vi "AnalyzeCommonTypeDefCallers.vi"() -> ()   [LabVIEW 2013, in "DiscoverCommonTypeDefCallers.lvlib"]
uses:
  DiscoverCommonTypeDefCallers.lvlib
panel:
  in  "Tab Control":enum32{"Tree View", "Table View"}(tab)
  in  "Dependent TypeDefs (Tree)":string(tree) caption="Dependent TypeDefs"
  out "Dependent TypeDefs (table)":string[][](table) caption="Dependent TypeDefs"
  in  "Application Reference":refnum<vi>
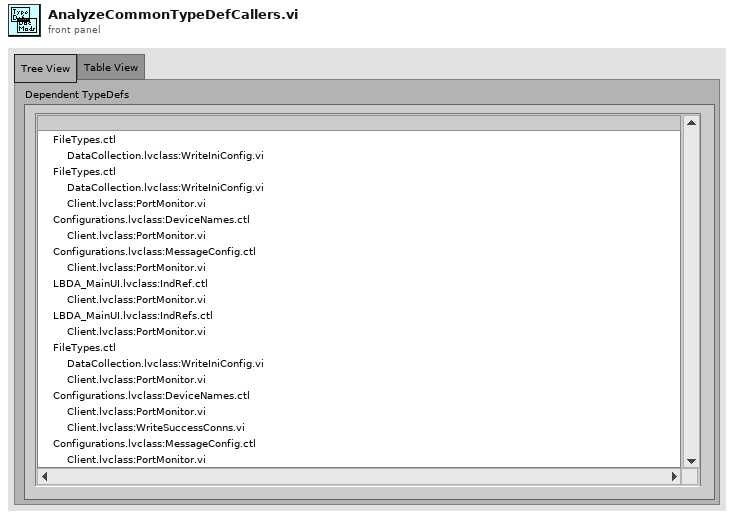
[diagram p1: front panel]
types:
  T1 = typedef "DiscoverCommonTypeDefCallers.lvlib/DependendentTypeDefwParents.ctl" = cluster{"TypeDef":string, "Non-strict / Strict":enum32{"Non-strict", "Strict"}, "Parent VIs":string[]}
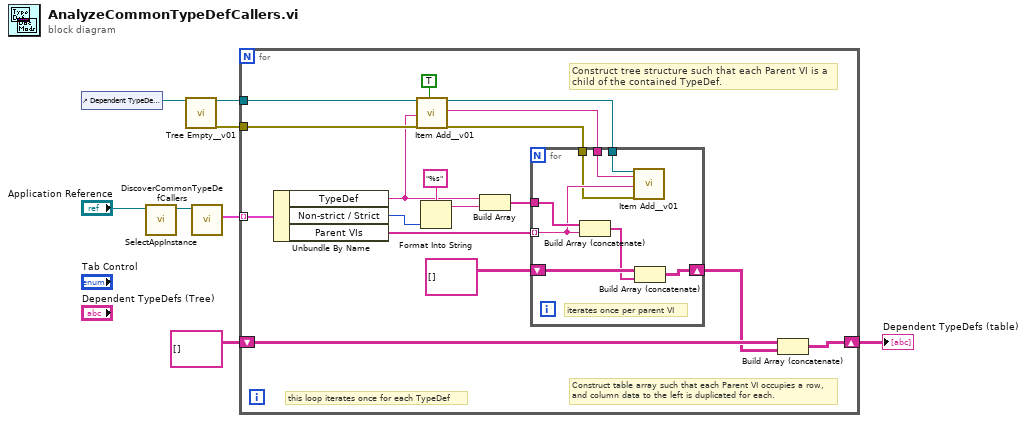
[diagram p0: block diagram]
diagram:
  n1 = control-ref of="Dependent TypeDefs (Tree)"() -> (w3:refnum<vi>)
  n2 = call "SelectAppInstance.vi"("Application Reference (in)"="Application Reference") -> ("Application Reference (out)"=w7:refnum<vi>)  [unwired: 8 in, 2 out]
  n3 = call <vilib>:"Tree Empty__v01.vi"("Tree Reference In"=w3) -> ("Tree Reference Out"=w2:refnum<vi>, "error out"=w1:errorcluster)  [unwired: 16 in, 1 out]
  n4 = call "DiscoverCommonTypeDefCallers.vi"("Application Reference"=w7) -> ("Dependendent TypeDefs wParents"=w6:T1[])  [unwired: 9 in, 1 out]
  n5 = for {
    tunnel: w6 -> [w25] mode=indexing
    shift-right: [w21] -> w4
    shift-left: string[][] [] -> [w20]
    tunnel: w2 -> [w14]
    tunnel: w1 -> [w13]
    # "Construct tree structure such that each Parent VI is a child of the contained TypeDef."
    # "this loop iterates once for each TypeDef"
    # "Construct table array such that each Parent VI occupies a row, and column data to the left is duplicated for each."
    n6 = Unbundle By Name(w25) -> ("TypeDef"=w12:string, "Non-strict / Strict"=w23:enum32{"Non-strict", "Strict"}, "Parent VIs"=w24:string[])
    n7 = call <vilib>:"Item Add__v01.vi"("Tree Reference In"=w14, "New Text Value"=w12, "error in (no error)"=w13, "Make Top Level Item"=TRUE) -> ("Tree Reference Out"=w11:refnum<vi>, "Created Tag"=w10:string, "error out"=w9:errorcluster)  [unwired: 13 in]
    n8 = Format Into String(format string="%s", w23) -> (resulting string=w18:string)  [unwired: 2 in, 1 out]
    n9 = Build Array(w12, w18) -> (w17:string[])
    n10 = for {
      tunnel: w24 -> [w27] mode=indexing
      shift-right: [w33] -> w19
      shift-left: string[][] [] -> [w32]
      tunnel: w17 -> [w31]
      tunnel: w11 -> [w29]
      tunnel: w10 -> [w28]
      tunnel: w9 -> [w26]
      # "iterates once per parent VI"
      n11 = Build Array (concatenate)(w31, w27) -> (w30:string[])
      n12 = call <vilib>:"Item Add__v01.vi"("Tree Reference In"=w29, "Parent Tag (Current)"=w28, "New Text Value"=w27, "error in (no error)"=w26) -> ()  [unwired: 13 in, 3 out]
      n13 = Build Array (concatenate)(w32, w30) -> (w33:string[][])
    }
    n14 = Build Array (concatenate)(w20, w19) -> (w21:string[][])
  }
  "Dependent TypeDefs (table)" <- w4
